vi "Open camera settings.vi"(8 "error in (no error)":errorcluster, 11 "IMAQdx Cam in":refnum<class "IMAQdx Cam.lvclass">) -> (0 "error out":errorcluster, 3 "IMAQdx Cam out":refnum<class "IMAQdx Cam.lvclass">)   [LabVIEW 2009, in "IMAQdx Cam.lvclass"]
uses:
  IMAQdx Cam.lvclass
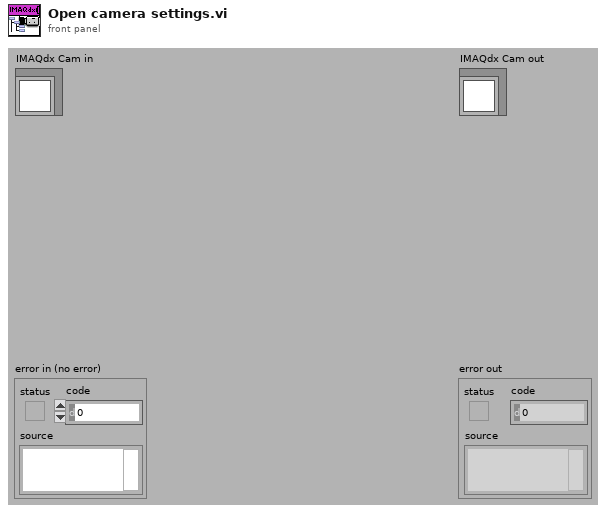
[diagram p1: front panel]
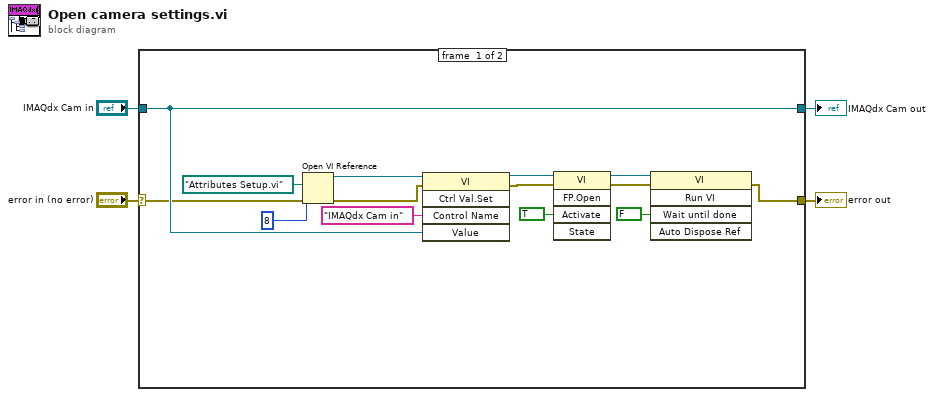
[diagram p0: block diagram]
diagram:
  n1 = case shown="No Error" "error in (no error)" {
    selector: "error in (no error)" -> [w13 w20]
    tunnel: [w10 w20] -> w3
    tunnel: [w15 w19] -> w1
    tunnel: "IMAQdx Cam in" -> [w15 w19]
    frame #0 {
      n2 = Open VI Reference(vi path=path "Attributes Setup.vi", options=8, error in (no error)=w13) -> (vi reference=w17:refnum<vi>, error out=w14:errorcluster)  [unwired: 3 in]
      n3 = invoke class="VI" method="Ctrl Val.Set"(reference=w17, error in=w14, "Control Name"="IMAQdx Cam in", "Value"=w15) -> (reference out=w12:refnum<vi>, error out=w7:errorcluster)  [unwired: 1 in, 3 out]
      n4 = invoke class="VI" method="FP.Open"(reference=w12, error in=w7, "Activate"=TRUE ("Activate?")) -> (reference out=w9:refnum<vi>, error out=w6:errorcluster)  [unwired: 2 in, 3 out]
      n5 = invoke class="VI" method="Run VI"(reference=w9, error in=w6, "Wait until done"=FALSE ("Wait Until Done")) -> (error out=w10:errorcluster)  [unwired: 2 in, 4 out]
    }
    frame #1 {
    }
  }
  "error out" <- w3
  "IMAQdx Cam out" <- w1
